vi "Kill Ninjas.vi"() -> ()   [LabVIEW 2012]
panel:
  in  "Previous Ninja\n Heading 2":dbl
  in  "Previous Ninja\n Y Position 2":dbl
  in  "Previous Ninja\n X Position 2":dbl
  in  "Previous Ninja \nHeading":dbl
  in  "Previous Ninja\n Y Position":dbl
  in  "Previous Ninja\n X Position":dbl
  in  "Ninja Heading":dbl
  in  "Ninja Y Position":dbl
  in  "Ninja X Position":dbl
  in  "Our Heading":dbl
  in  "Our Y Position":dbl
  in  "Our X Position":dbl
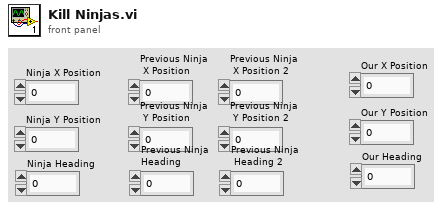
[diagram p1: front panel]
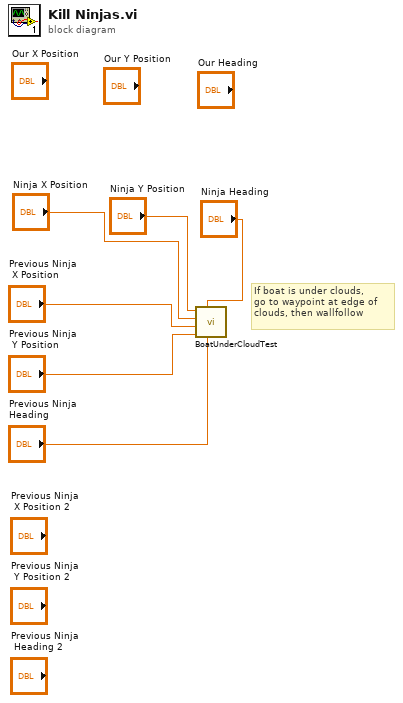
[diagram p0: block diagram]
diagram:
  # "If boat is under clouds, \ngo to waypoint at edge of \nclouds, then wallfollow"
  n1 = call "BoatUnderCloudTest.vi"("HDG 2"="Previous Ninja \nHeading", "HDG"="Ninja Heading", "Y 2"="Previous Ninja\n Y Position", "X 2"="Previous Ninja\n X Position", "X"="Ninja X Position", "Y"="Ninja Y Position") -> ()  [unwired: 1 out]
